vi "Page_ReplaceProject.vi"(8 "error in (no error)":errorcluster, 11 "Configuration Paths in":T1) -> (0 "error out":errorcluster, 3 "Configuration Paths out":T1)   [LabVIEW 2010]
uses:
  Config cluster.ctl
panel:
  out "Current Project":string
  in  "Delete":bool
  in  "OK":bool
  in  "Selected Project Files":i32(listbox)
  in  "Configuration Files":i32(listbox)=-1
  in  "Cancel":bool
  in  "Replace with":bool
  in  "Mode":enum16{"MIL", "HIL", "XiL"}(ring)
  # "1) Choose the type of test to be performed"
  # "2) Select the configuration files that will be used in the test(s)"
  # "Available Project Files"
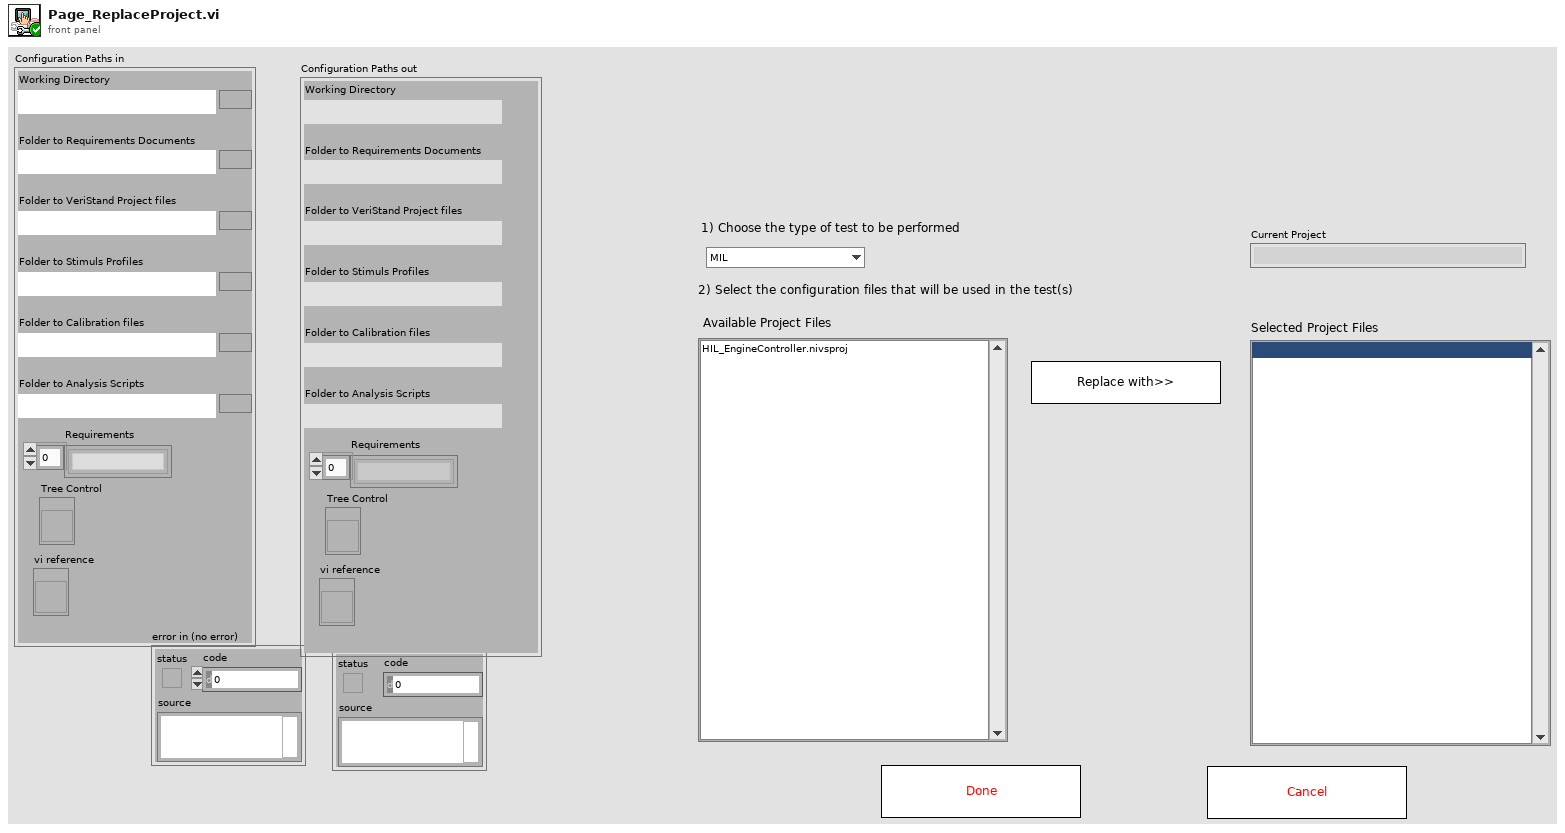
[diagram p1: front panel]
types:
  T1 = typedef "Config cluster.ctl" = cluster{"Working Directory":path, "Folder to Requirements Documents":path, "Folder to VeriStand Project files":path, "Folder to Stimuls Profiles":path, "Folder to Calibration files":path, "Folder to Analysis Scripts":path, "Requirements":string[], "Tree Control":refnum<vi>, "vi reference":refnum<vi>}
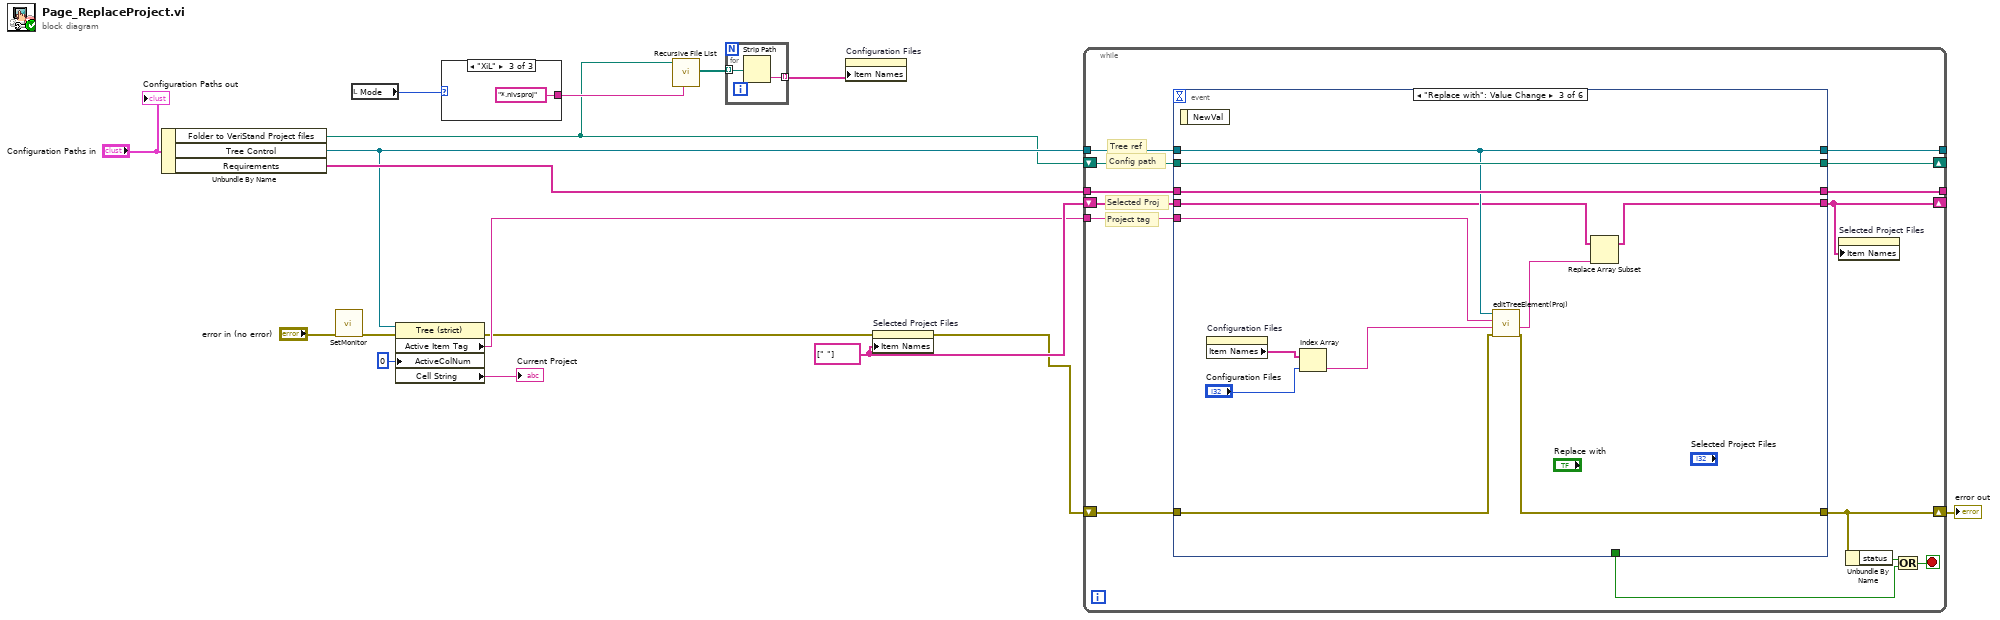
[diagram p0: block diagram]
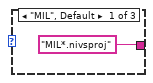
[diagram p2: hidden frame]
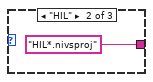
[diagram p3: hidden frame]
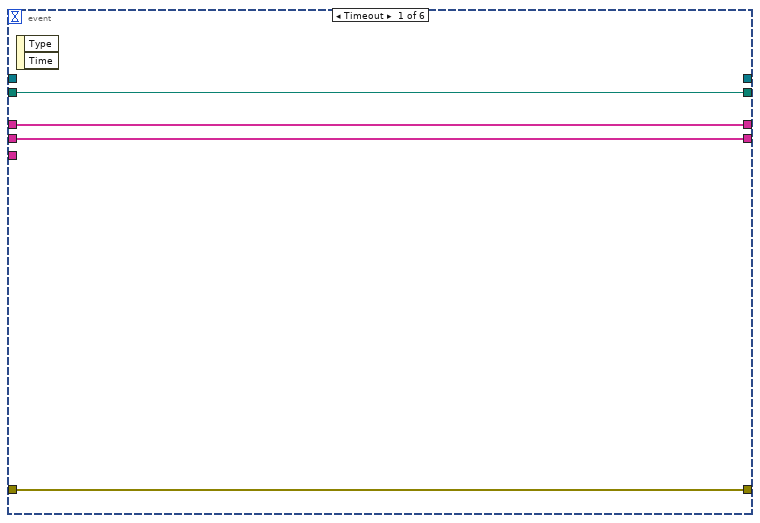
[diagram p4: hidden frame]
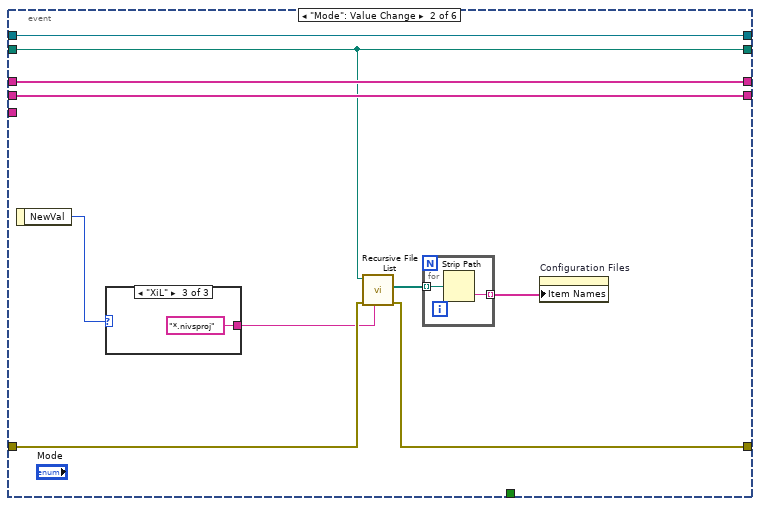
[diagram p5: hidden frame]
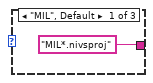
[diagram p6: hidden frame]
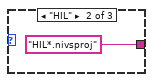
[diagram p7: hidden frame]
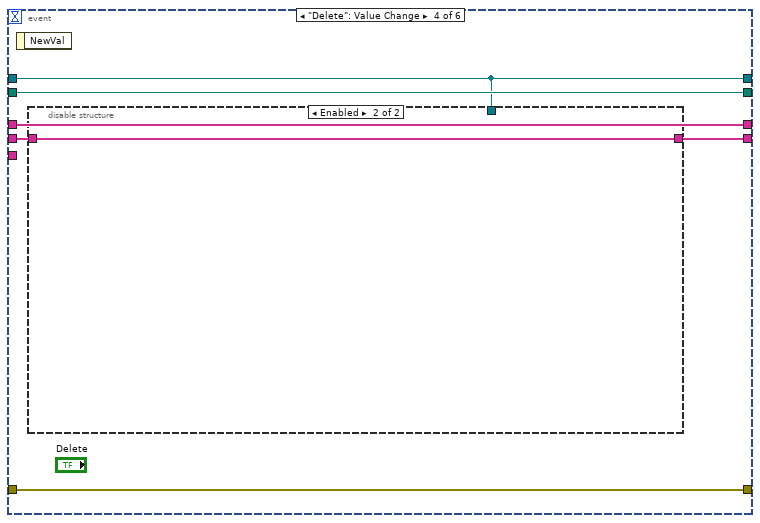
[diagram p8: hidden frame]
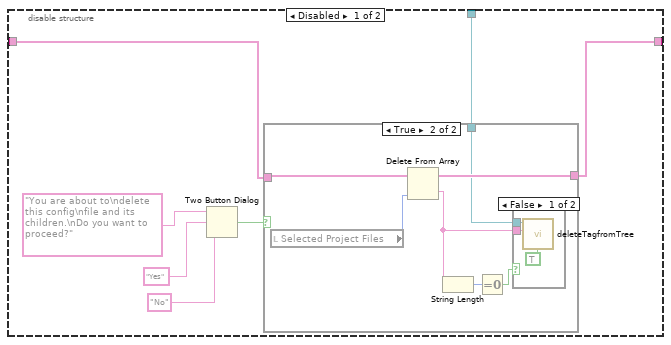
[diagram p9: hidden frame]
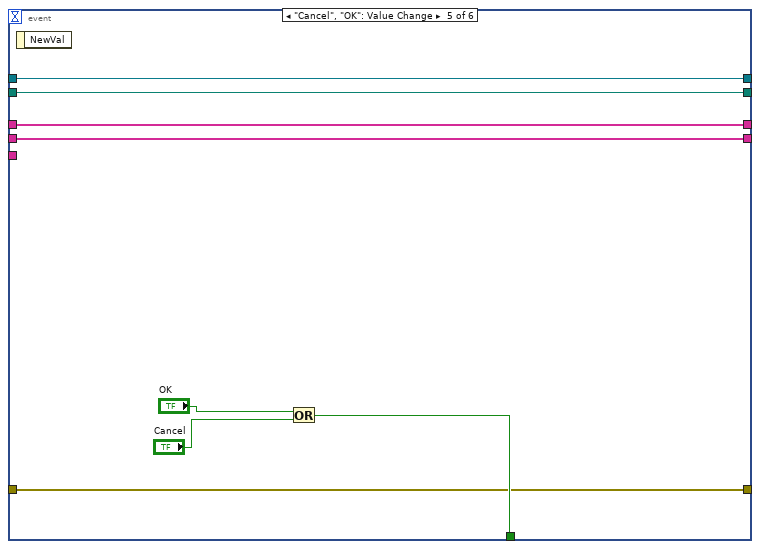
[diagram p12: hidden frame]
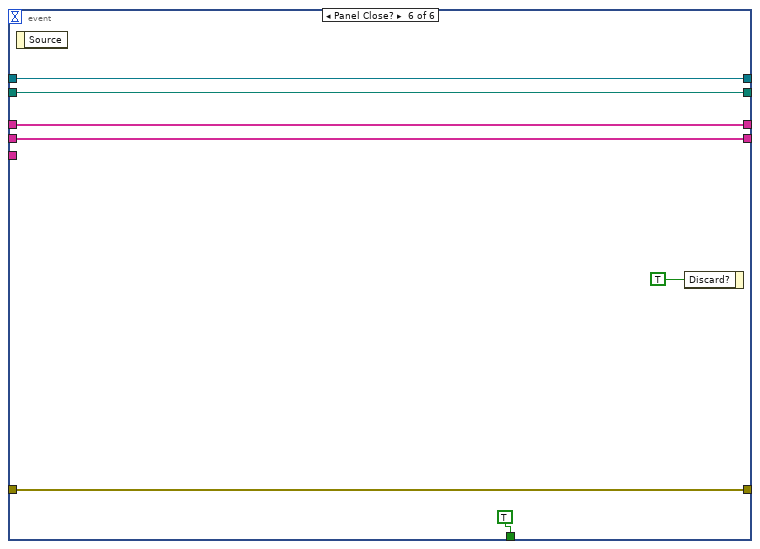
[diagram p13: hidden frame]
diagram:
  w14 = string[] [" "]
  n1 = Unbundle By Name("Configuration Paths in") -> ("Folder to VeriStand Project files"=w7:path, "Tree Control"=w15:refnum<vi>, "Requirements"=w16:string[])
  n2 = call "SetMonitor.vi"("error in (no error)"="error in (no error)") -> ("error out"=w6:errorcluster)  [unwired: 9 in, 1 out]
  n3 = local read "Mode"() -> (w8:enum16{"MIL", "HIL", "XiL"})
  n4 = property class="Tree (strict)"(reference=w15, error in=w6, "ActiveColNum"=0 ("Active Cell:Active Column Number")) -> (error out=w4:errorcluster, "Active Item Tag"=w12:string, "Cell String"=→"Current Project":string)  [unwired: 1 out]
  n5 = case shown="\"XiL\"" w8 {
    tunnel: ["MIL*.nivsproj" ("name or relative path") "HIL*.nivsproj" ("name or relative path") "*.nivsproj" ("name or relative path")] -> w9
    frame "MIL", Default {
    }
    frame "HIL" {
    }
    frame "XiL" {
    }
  }
  n6 = call <vilib>:"Recursive File List.vi"("pattern"=w9, "Folder Path"=w7) -> ("All Files in Dir"=w11:path[])  [unwired: 5 in, 4 out]
  n7 = for {
    tunnel: w11 -> [w22] mode=indexing
    tunnel: [w21] -> w10 mode=indexing
    n8 = Strip Path(path=w22) -> (name=w21:string)  [unwired: 1 out]
  }
  n9 = property on="Configuration Files" class="LstBox (strict)"("Item Names"=w10) -> ()  [unwired: 2 in, 2 out]
  n10 = property on="Selected Project Files" class="LstBox (strict)"(error in=w4, "Item Names"=w14) -> (error out=w3:errorcluster)  [unwired: 1 in, 1 out]
  n11 = while {
    tunnel: w15 -> [w36]
    tunnel: w16 -> [w35]
    shift-right: [w34] -> _
    shift-left: w7 -> [w33]
    tunnel: [w32] -> _
    tunnel: [w30] -> _
    shift-right: [w27] -> w13
    shift-left: w3 -> [w28]
    tunnel: w12 -> [w23]
    shift-right: [w29] -> _
    shift-left: w14 -> [w31]
    stop <- w24 stop-if-true
    # "Project tag"
    # "Selected Proj"
    # "Tree ref"
    # "Config path"
    n12 = event shown="[2] \"Replace with\": Value Change" {
      selector: _ -> [_ _ _ _ _ _]
      dyn-events: _ -> [_ _ _ _ _ _]
      timeout: _ -> [_ _ _ _ _ _]
      tunnel: [_ _ _ _ w97 TRUE] -> w25
      tunnel: [w40 w41 w66 w72 w93 w103] -> w34
      tunnel: w36 -> [_ w48 w62 w69 w92 w102]
      tunnel: w35 -> [w38 w45 w65 w71 w95 w105]
      tunnel: w33 -> [w40 w41 w66 w72 w93 w103]
      tunnel: [_ w48 w62 w69 w92 w102] -> w32
      tunnel: w31 -> [w37 w44 w58 w70 w94 w104]
      tunnel: [w37 w44 w57 w68 w94 w104] -> w29
      tunnel: [w38 w45 w65 w71 w95 w105] -> w30
      tunnel: w28 -> [w39 w47 w60 w67 w96 w106]
      tunnel: [w39 w46 w59 w67 w96 w106] -> w27
      tunnel: w23 -> [_ _ w61 _ _ _]
      event Timeout {
        n13 = event-data() -> ()  [unwired: 1 in, 2 out]
      }
      event "Mode": Value Change {
        n14 = event-data() -> ("NewVal"=w43:enum16{"MIL", "HIL", "XiL"})  [unwired: 1 in]
        n15 = case shown="\"XiL\"" w43 {
          tunnel: ["MIL*.nivsproj" ("name or relative path") "HIL*.nivsproj" ("name or relative path") "*.nivsproj" ("name or relative path")] -> w42
          frame "MIL", Default {
          }
          frame "HIL" {
          }
          frame "XiL" {
          }
        }
        n16 = call <vilib>:"Recursive File List.vi"("pattern"=w42, "error in (no error)"=w47, "Folder Path"=w41) -> ("error out"=w46:errorcluster, "All Files in Dir"=w50:path[])  [unwired: 4 in, 3 out]
        n17 = for {
          tunnel: w50 -> [w55] mode=indexing
          tunnel: [w54] -> w49 mode=indexing
          n18 = Strip Path(path=w55) -> (name=w54:string)  [unwired: 1 out]
        }
        n19 = property on="Configuration Files" class="LstBox (strict)"("Item Names"=w49) -> ()  [unwired: 2 in, 2 out]
      }
      event "Replace with": Value Change {
        n20 = event-data() -> ()  [unwired: 1 in, 1 out]
        n21 = property on="Configuration Files" class="LstBox (strict)"() -> ("Item Names"=w64:string[])  [unwired: 2 in, 2 out]
        n22 = Index Array(array=w64, index="Configuration Files") -> (element=w56:string)
        n23 = call "editTreeElement(Proj).vi"("error in (no error)"=w60, "Project File"=w56, "Active Item:Tag"=w61, "Tree Control in"=w62) -> ("error out"=w59:errorcluster)  [unwired: 7 in]
        n24 = Replace Array Subset(array=w58, new element=w56) -> (w57:string[])  [unwired: 1 in]
      }
      event "Delete": Value Change {
        n25 = event-data() -> ()  [unwired: 1 in, 1 out]
        n26 = disable-structure shown="Enabled" {
          disable-tunnel: w70 -> [w76 w91]
          disable-tunnel: w69 -> [w75 _]
          disable-tunnel: [w74 w91] -> w68
          frame Disabled {
            n27 = Two Button Dialog(message="You are about to\ndelete this config\nfile and its children.\nDo you want to proceed?", 1:"No" ("F button name (\"Cancel\")"), 2:"Yes" ("T button name (\"OK\")")) -> (T button?=w79:bool)
            n28 = case shown="True" w79 {
              tunnel: w76 -> [w80 w87]
              tunnel: [w80 w86] -> w74
              tunnel: w75 -> [_ w85]
              frame False {
              }
              frame True {
                n29 = local read "Selected Project Files"() -> (w84:i32)
                n30 = Delete From Array(array=w87, index=w84) -> (deleted portion=w83:string, array with subset deleted=w86:string[])  [unwired: 1 in]
                n31 = String Length(string=w83) -> (length=w82:i32)
                n32 = Equal To 0?(x=w82) -> (x = 0?=w81:bool)
                n33 = case shown="False" w81 {
                  tunnel: w85 -> [w90 _]
                  tunnel: w83 -> [w88 _]
                  frame False {
                    n34 = call "deleteTagfromTree.vi"("Delete Children?"=TRUE, "Tag"=w88, "Tree Ref"=w90) -> ()  [unwired: 7 in, 2 out]
                  }
                  frame True {
                  }
                }
              }
            }
          }
          frame Enabled {
          }
        }
      }
      event "Cancel", "OK": Value Change {
        n35 = event-data() -> ()  [unwired: 1 in, 1 out]
        n36 = Or(x="OK", y="Cancel") -> (x .or. y?=w97:bool)
      }
      event Panel Close? {
        n37 = event-data() -> ()  [unwired: 1 in, 1 out]
        n38 = event-data("Discard?"=TRUE) -> ()  [unwired: 1 in, 1 out]
      }
    }
    n39 = property on="Selected Project Files" class="LstBox (strict)"("Item Names"=w29) -> ()  [unwired: 2 in, 2 out]
    n40 = Unbundle By Name(w27) -> ("status"=w26:bool)
    n41 = Or(x=w26, y=w25) -> (x .or. y?=w24:bool)
  }
  "error out" <- w13
  "Configuration Paths out" <- "Configuration Paths in"
